vi "Parse Groups Part 2.vi"(11 "Input":string="???.### 1,1,3\n.??..??...?##. 1,1,3\n?#?#?#?#?#?#?#? 1,3,1,6\n????.#...#... 4,1,1\n????.######..#####. 1,6,5\n?###???????? 3,2,1") -> (2 "Counts":i64[][](array[numeric]), 3 "Groups":refnum<class "Group.lvclass">[](array[class]))   [LabVIEW 2021]
uses:
  Group.lvclass
  Helpers/Helpers.lvlib
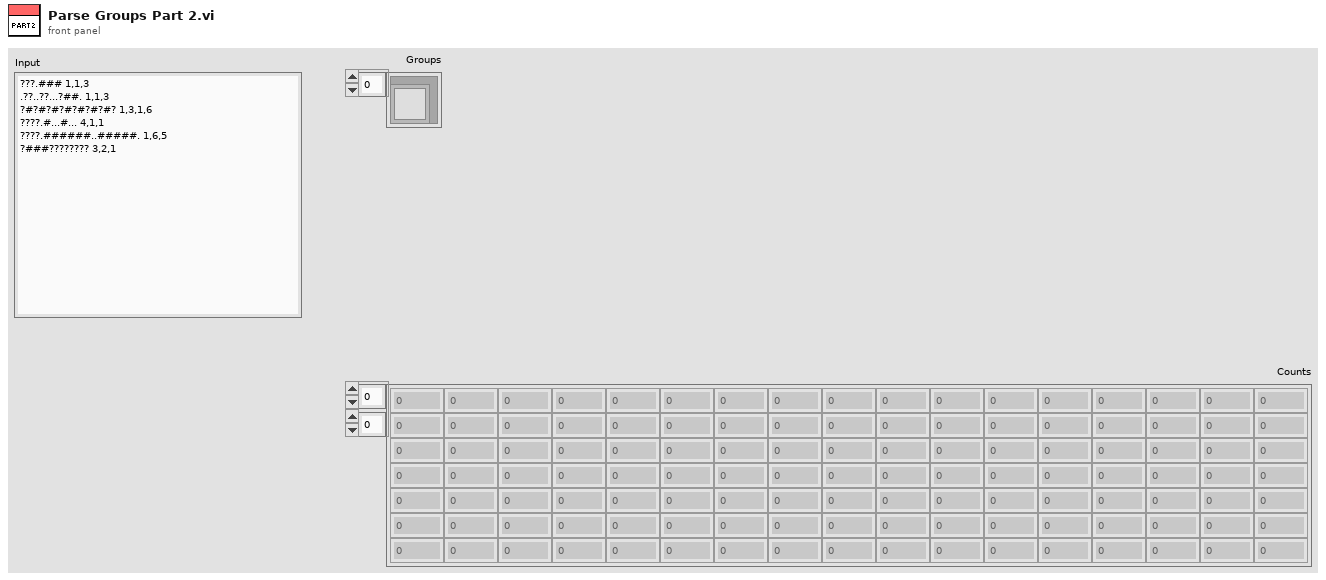
[diagram p1: front panel]
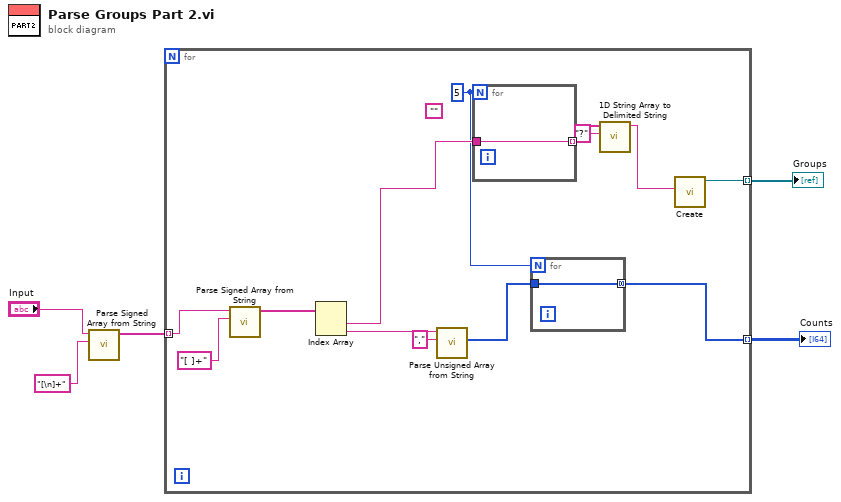
[diagram p0: block diagram]
diagram:
  n1 = call "Parse Signed Array from String.vi"("Delimiter regex"="[\n]+", "Input"="Input") -> ("Parsed Array"=w2:string[])  [unwired: 8 in, 1 out]
  n2 = for {
    tunnel: [w14] -> w5 mode=indexing
    tunnel: w2 -> [w13] mode=indexing
    tunnel: [w10] -> w1 mode=indexing
    w9 = 5
    (unwired) "" ("element")
    n3 = call "Parse Signed Array from String.vi"("Delimiter regex"="[ ]+", "Input"=w13) -> ("Parsed Array"=w17:string[])  [unwired: 8 in, 1 out]
    n4 = Index Array(array=w17) -> (element #1=w12:string, element #2=w16:string)  [unwired: 2 in]
    n5 = call "Parse Unsigned Array from String.vi"("Delimiter regex"=",", "Input"=w16) -> ("Parsed U64 Array"=w11:u64[])  [unwired: 8 in, 1 out]
    n6 = for {
      N: w9 -> [_]
      tunnel: w12 -> [w20]
      tunnel: [w20] -> w8 mode=indexing
    }
    n7 = for {
      N: w9 -> [_]
      tunnel: w11 -> [w19]
      tunnel: [w19] -> w10 mode=concatenating
    }
    n8 = call <vilib>:"1D String Array to Delimited String.vi"("delimiter"="?", "string array"=w8) -> ("delimited string"=w6:string)  [unwired: 9 in]
    n9 = call "Create.vi"("Input"=w6) -> ("Group Out"=w14:refnum<class "Group.lvclass">)  [unwired: 9 in, 1 out]
  }
  "Groups" <- w5
  "Counts" <- w1
